vi "TimedDoor2_Create.vi"(0 "reference in":refnum<class "TimedDoor2.lvclass">, 5 "error in (no error)":errorcluster) -> (14 "reference out":refnum<class "TimedDoor2.lvclass">, 19 "error out":errorcluster)   [LabVIEW 2020, in "TimedDoor2.lvclass"]
uses:
  TimedDoor2.lvclass
  C:/Projects/DesignPatterns_Trunk/Timer/Door_class/Door.lvclass
  Door_class/Door.lvclass
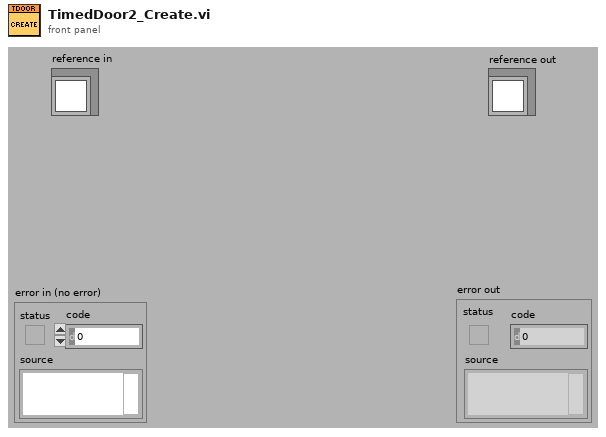
[diagram p1: front panel]
types:
  T1 = typedef "TimedDoor2.lvclass/ObjectAttributes.ctl" = cluster{"Attribute1":dbl}
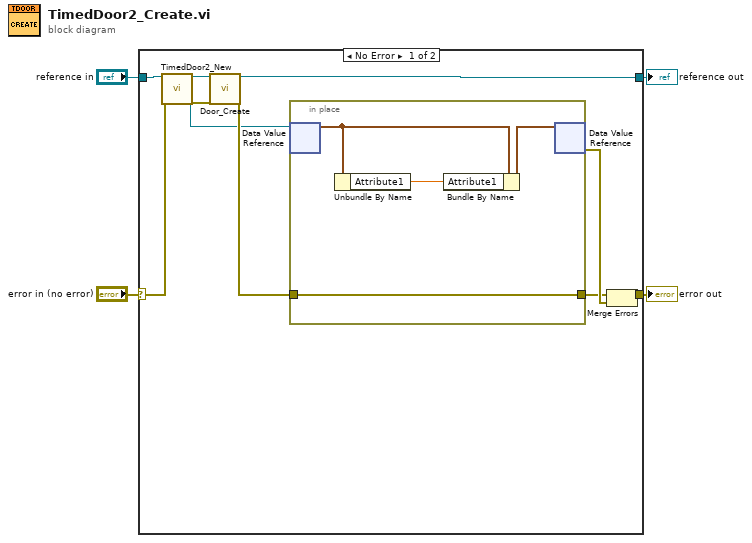
[diagram p0: block diagram]
diagram:
  n1 = case shown="No Error" "error in (no error)" {
    selector: "error in (no error)" -> [w8 w20]
    tunnel: [w10 w20] -> w3
    tunnel: "reference in" -> [w9 w19]
    tunnel: [w14 w19] -> w1
    frame No Error {
      n2 = call "TimedDoor2_New.vi"("reference in"=w9, "error in (no error)"=w8) -> ("reference out"=w7:refnum<class "TimedDoor2.lvclass">, "DVRRefOut"=w5:refnum<data-value>, "error out"=w6:errorcluster)  [unwired: 14 in, 1 out]
      n3 = call "Door_Create.vi"("reference in"=w7, "error in (no error)"=w6) -> ("reference out"=w14:refnum<class "TimedDoor2.lvclass">, "error out"=w12:errorcluster)  [unwired: 16 in]
      n4 = in-place {
        in-place-border: w12 -> [w15]
        in-place-border: [w15] -> w11
        n5 = in-place-dvr #1(w5) -> (w17:T1)  [unwired: 1 out]
        n6 = Unbundle By Name(w17) -> ("Attribute1"=w16:dbl)
        n7 = Bundle By Name(cluster=w17, "Attribute1"=w16) -> (w18:T1)
        n8 = in-place-dvr #1(w18) -> (w13:errorcluster)  [unwired: 1 out]
      }
      n9 = Merge Errors(w11, w13) -> (w10:errorcluster)
    }
    frame Error {
      # "VI-TechBaseTemplate_Simple_4x4x4"
    }
  }
  "error out" <- w3
  "reference out" <- w1
